vi "TabLatch.vi"(8 "Switch State":bool, 11 "Controls Tab":u32) -> (0 "Switch State":bool)   [LabVIEW 2016]
panel:
  # "Tab-switched controls use an RS NOR latch \nto toggle off when not on the correct pane\nand remain off until switched on again."
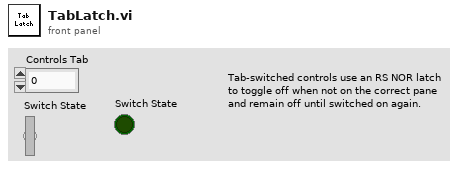
[diagram p1: front panel]
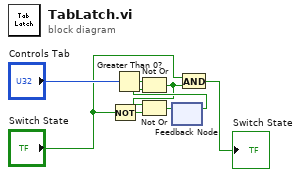
[diagram p0: block diagram]
diagram:
  n1 = Not(x="Switch State") -> (.not. x?=w5:bool)
  n2 = Greater Than 0?(x="Controls Tab") -> (x > 0?=w7:bool)
  n3 = feedback #1() -> (w6:bool)  [unwired: 1 in]
  n4 = Not Or(1:w6, 2:w7) -> (0:w4:bool)
  n5 = Not Or(1:w5, 2:w4) -> (0:w8:bool)
  n6 = feedback-in #1(w8) -> ()
  n7 = And(x="Switch State", y=w4) -> (x .and. y?=→"Switch State":bool)
